vi "testLoopback.vi"(8 "error in (no error)":errorcluster, 11 "TestCase in":refnum<class "SystemTestCase.lvclass">) -> (0 "error out":errorcluster, 3 "TestCase out":refnum<class "SystemTestCase.lvclass">)   [LabVIEW 2018, in "SystemTestCase.lvclass"]
uses:
  SystemTestCase.lvclass
  C:/Users/mbilyk/Documents/github/ni/niveristand-custom-device-testing-tools/VeriStandTestCase/VeriStandTestCase.lvclass
  <vilib>/addons/_JKI Toolkits/VI Tester/TestCase.llb/TestCase.lvclass
  github/ni/niveristand-custom-device-testing-tools/VeriStandTestCase/VeriStandTestCase.lvclass
  C:/Program Files (x86)/National Instruments/LabVIEW 2018/vi.lib/addons/_JKI Toolkits/VI Tester/TestCase.llb/TestCase.lvclass
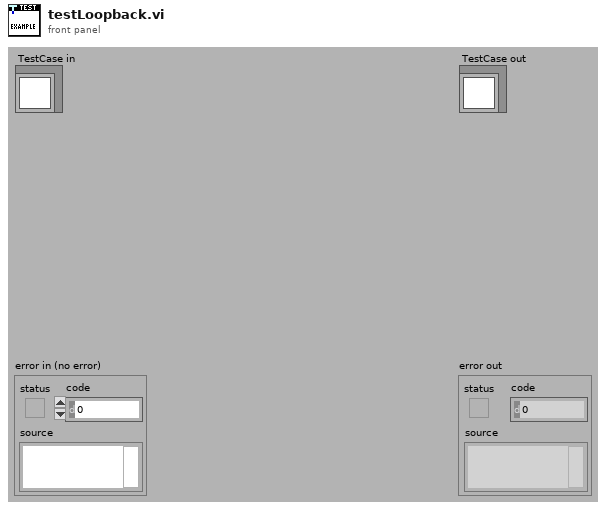
[diagram p1: front panel]
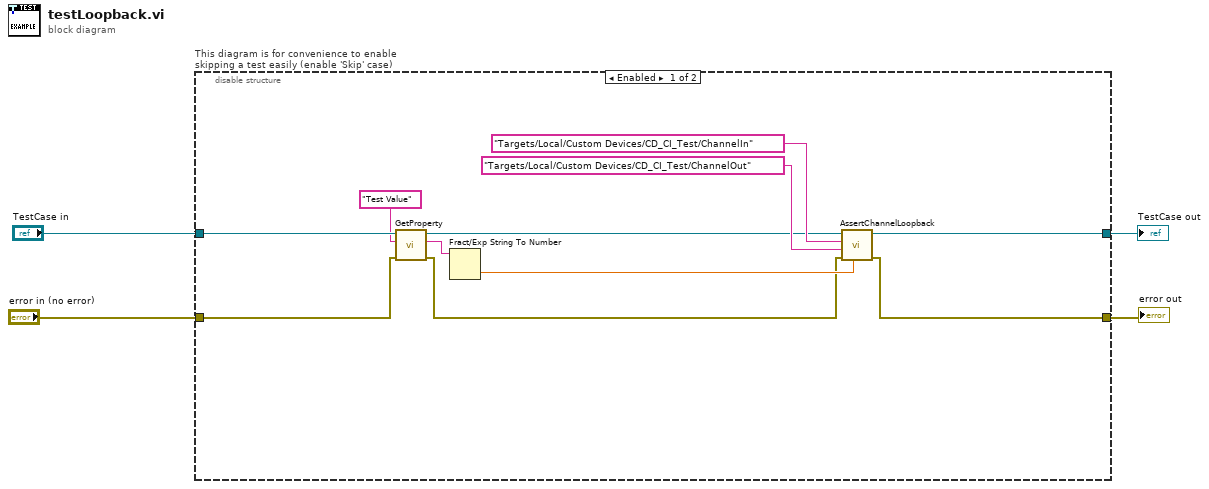
[diagram p0: block diagram]
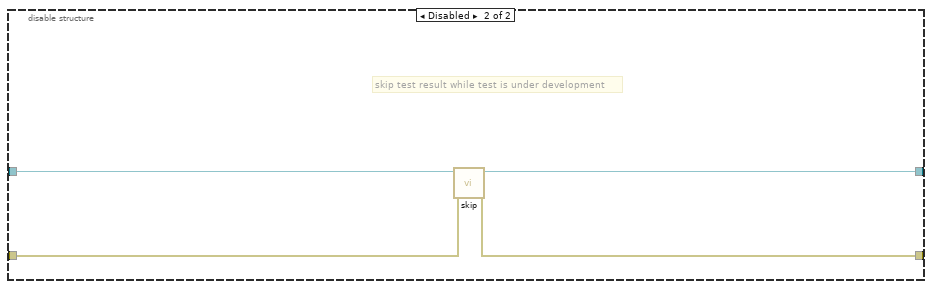
[diagram p2: hidden frame]
diagram:
  n1 = disable-structure "This diagram is for convenience to enable skipping a test easily (enable 'Skip' case)" shown="Enabled" {
    disable-tunnel: "TestCase in" -> [w15 w19]
    disable-tunnel: [w6 w17] -> w1
    disable-tunnel: [w5 w18] -> w3
    disable-tunnel: "error in (no error)" -> [w14 w16]
    frame Enabled {
      n2 = call "GetProperty.vi"("error in (no error)"=w14, "key"="Test Value", "VeriStandTestCase in"=w15) -> ("error out"=w7:errorcluster, "value"=w12:string, "VeriStandTestCase out"=w8:refnum<class "SystemTestCase.lvclass">)  [unwired: 6 in]
      n3 = Fract/Exp String To Number(string=w12) -> (number=w11:dbl)  [unwired: 3 in, 1 out]
      n4 = call "AssertChannelLoopback.vi"("Value"=w11, "error in (no error)"=w7, "Read Channel"="Targets/Local/Custom Devices/CD_CI_Test/ChannelOut" ("key"), "Write Channel"="Targets/Local/Custom Devices/CD_CI_Test/ChannelIn" ("key"), "VeriStand Test Case in"=w8) -> ("error out"=w5:errorcluster, "VeriStand Test Case out"=w6:refnum<class "SystemTestCase.lvclass">)  [unwired: 5 in]
    }
    frame Disabled {
      # "skip test result while test is under development"
      n5 = call <vilib>:"skip.vi"("error in (no error)"=w16, "TestCase in"=w19) -> ("error out"=w18:errorcluster, "TestCase out"=w17:refnum<class "SystemTestCase.lvclass">)  [unwired: 8 in]
    }
  }
  "error out" <- w3
  "TestCase out" <- w1
